vi "Instantiate.vi"(0 "scripts manager in":refnum<class "scripts manager.lvclass">, 11 "error in (no error)":errorcluster) -> (4 "scripts manager out":refnum<class "scripts manager.lvclass">, 15 "error out":errorcluster)   [LabVIEW 2016, in "scripts manager.lvclass"]
uses:
  scripts manager.lvclass
  scripts manager.lvclass/scripts manager.ctl
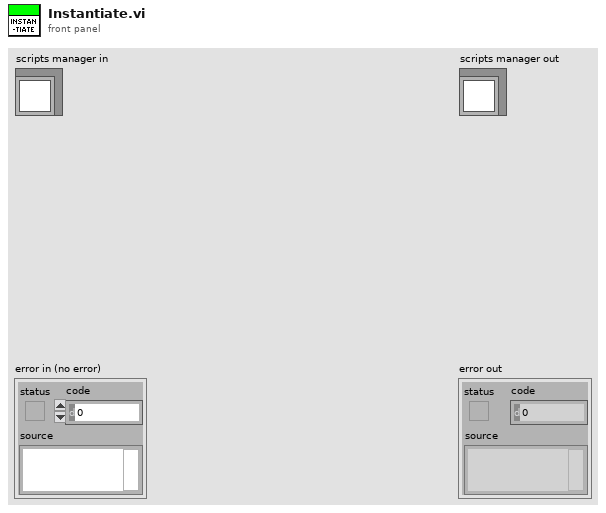
[diagram p1: front panel]
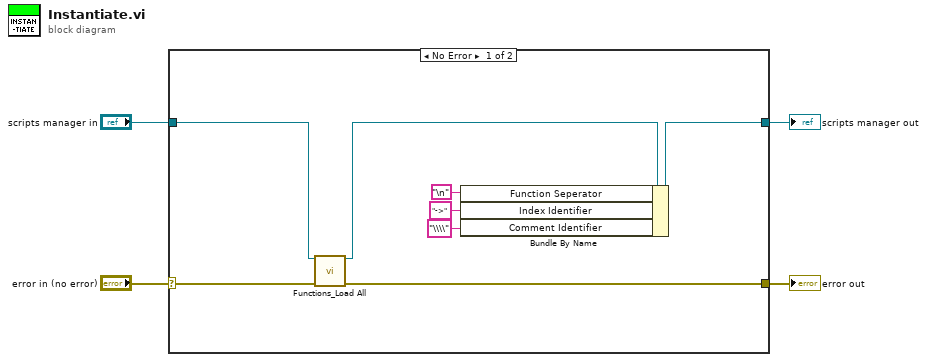
[diagram p0: block diagram]
diagram:
  n1 = case shown="No Error" "error in (no error)" {
    selector: "error in (no error)" -> [w8 w14]
    tunnel: [w7 w14] -> w3
    tunnel: [w12 w13] -> w1
    tunnel: "scripts manager in" -> [w6 w13]
    frame No Error {
      n2 = call-dynamic "Functions_Load All.vi"("scripts manager in"=w6, "error in (no error)"=w8) -> ("scripts manager out"=w5:refnum<class "scripts manager.lvclass">, "error out"=w7:errorcluster)  [unwired: 12 in]
      n3 = Bundle By Name(cluster=w5, "Function Seperator"="\n", "Index Identifier"="->" ("Function Rules.Index Identifier"), "Comment Identifier"="\\\\" ("Function Rules.Comment Identifier")) -> (w12:refnum<class "scripts manager.lvclass">)
    }
    frame Error {
    }
  }
  "error out" <- w3
  "scripts manager out" <- w1
